vi "Initialize.vi"(8 "Error In":errorcluster, 10 "Folder Path":path, 11 "Plugin Framework In":refnum<class "File Parsing Interface.lvclass">) -> (0 "Error Out":errorcluster, 3 "File Parsing Interface out":refnum<class "File Parsing Interface.lvclass">)   [LabVIEW 2018, in "File Parsing Interface.lvlib" / "File Parsing Interface.lvclass"]
uses:
  File Parsing Interface.lvclass
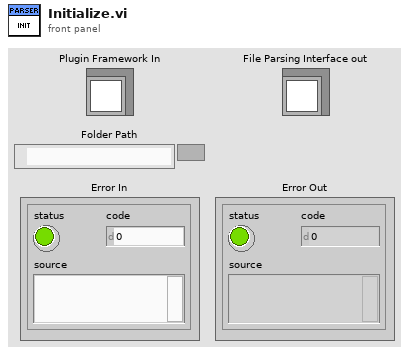
[diagram p1: front panel]
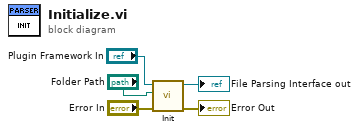
[diagram p0: block diagram]
diagram:
  n1 = call-dynamic "Init.vi"("Error In"="Error In", "Folder Path"="Folder Path", "Plugin Framework In"="Plugin Framework In") -> ("Error Out"=→"Error Out":errorcluster, "Factory Plugin Framework out"=→"File Parsing Interface out":refnum<class "File Parsing Interface.lvclass">)  [unwired: 7 in]
